vi "Finish.vi"   [LabVIEW 2019]
doc: "This VI is called just before exiting. It is expected to close I/O refnum, save collected data, etc."
uses:
  <vilib>/Rock Robotics/WPI/Utilities/WPI_GetSetVariantRefNum.vi
types:
  T1 = typedef "WPI_JoystickDevRef.ctl" = cluster{"Device":T2}
  T2 = typedef "WPI_JoystickDeviceEnum.ctl" = enum16{"USB 0", "USB 1", "USB 2", "USB 3", "USB 4", "USB 5"}
  T3 = typedef "WPI_CameraDevRef.ctl" = cluster{"Camera Address":string, "CameraStatus":errorcluster}
  T4 = typedef "WPI_SolenoidDevRef.ctl" = cluster{"DevStatus":errorcluster, "Pneumatics Control Module":u8, "Forward Solenoid Channel":T5, "Reverse Solenoid Channel":T5}
  T5 = typedef "WPI_SolenoidChannel.ctl" = enum8{"Solenoid 0", "Solenoid 1", "Solenoid 2", "Solenoid 3", "Solenoid 4", "Solenoid 5", "Solenoid 6", "Solenoid 7", "Invalid"}
  T6 = typedef "WPI_CompressorDevRef.ctl" = cluster{"DevStatus":errorcluster, "Pneumatics Control Module":u8}
  T7 = typedef "WPI_RobotDriveDevRef.ctl" = cluster{"DevStatus":errorcluster, "Motors[]":T8[], "Square Inputs":bool, "Max Output":dbl}
  T8 = typedef "WPI_MotorControlDeviceRef.ctl" = cluster{"DeviceStatus":errorcluster, "Type":T9, "PWM":cluster{"PWM Channel":T10, "DeadBand":T11}, "CAN":cluster{"Device Number":u8, "SetOutput VI Ref":variant, "GetOutput VI Ref":variant, "Enable VI Ref":variant, "Disable VI Ref":variant, "Data":variant}, "Invert":bool, "DIO PWM":cluster{"PWM \"Enable\" Channel":T10, "DIOChannel":T12, "PWM Rate":dbl}}
  T9 = typedef "WPI_MotorControlType.ctl" = enum16{"PWM", "CAN", "DIO PWM"}
  T10 = typedef "FPGA_DIOPWMChannel.ctl" = enum8{"PWM 0", "PWM 1", "PWM 2", "PWM 3", "PWM 4", "PWM 5", "PWM 6", "PWM 7", "PWM 8", "PWM 9", "PWM MXP 0", "PWM MXP 1", "PWM MXP 2", "PWM MXP 3", "PWM MXP 4", "PWM MXP 5", "PWM MXP 6", "PWM MXP 7", "PWM MXP 8", "PWM MXP 9", "Invalid"}
  T11 = typedef "WPI_PWMDeadband.ctl" = cluster{"Name":string, "maxPositivePwm":i32, "minPositivePwm":i32, "centerPwm":i32, "maxNegativePwm":i32, "minNegativePwm":i32, "angularRange":u16}
  T12 = typedef "FPGA_DIOChannel.ctl" = enum8{"DIO 0", "DIO 1", "DIO 2", "DIO 3", "DIO 4", "DIO 5", "DIO 6", "DIO 7", "DIO 8", "DIO 9", "DIO MXP 0", "DIO MXP 1", "DIO MXP 2", "DIO MXP 3", "DIO MXP 4", "DIO MXP 5", "DIO MXP 6", "DIO MXP 7", "DIO MXP 8", "DIO MXP 9", "DIO MXP 10", "DIO MXP 11", "DIO MXP 12", "DIO MXP 13", "DIO MXP 14", "DIO MXP 15", "SPI Port CS1", "SPI Port CS2", "SPI Port CS3", "SPI Port MISO", "SPI Port MOSI", "Invalid"}
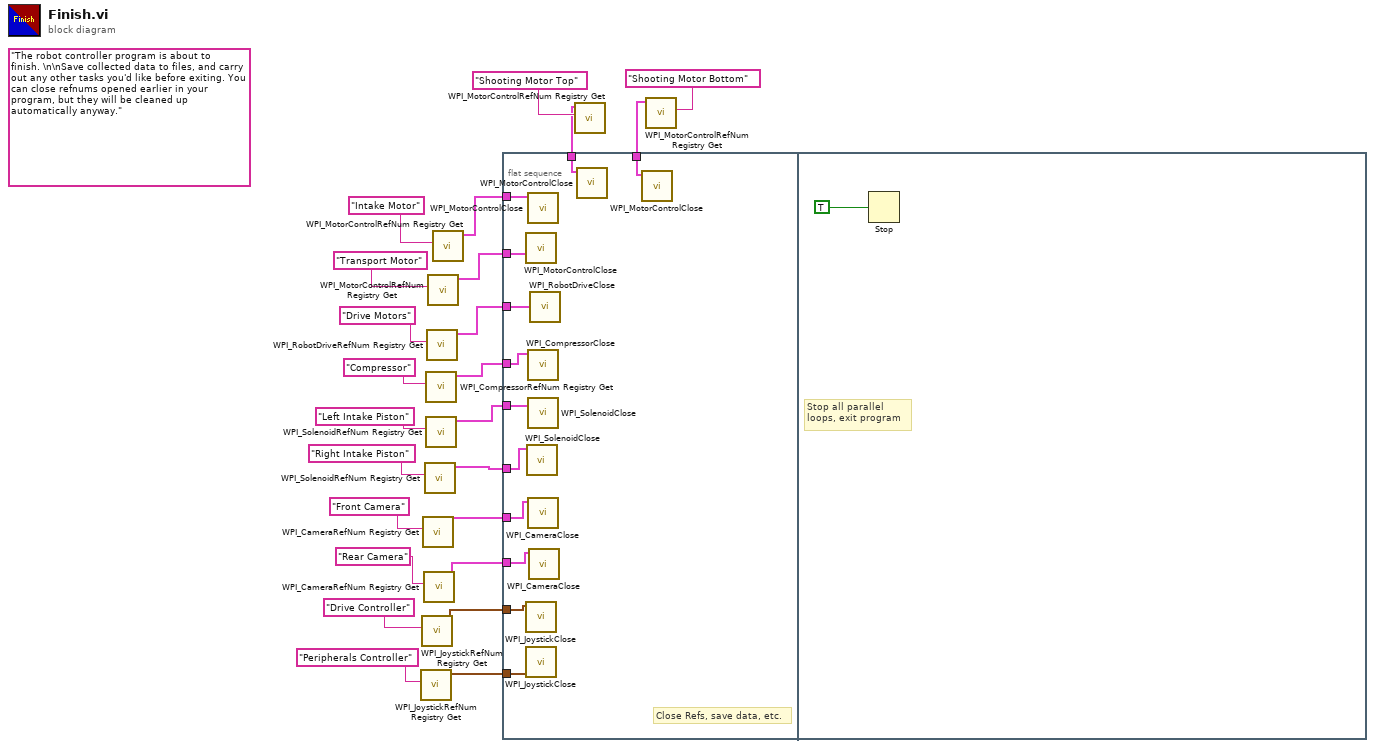
[diagram p0: block diagram]
diagram:
  (unwired) "The robot controller program is about to finish. \n\nSave collected data to files, and carry out any other tasks you'd like before exiting. You can close refnums opened earlier in your program, but they will be cleaned up automatically anyway."
  n1 = call <vilib>:"WPI_JoystickRefNum Registry Get.vi"("refnum name"="Peripherals Controller") -> ("JoystickDevRef"=w5:T1)  [unwired: 9 in, 1 out]
  n2 = call <vilib>:"WPI_JoystickRefNum Registry Get.vi"("refnum name"="Drive Controller") -> ("JoystickDevRef"=w6:T1)  [unwired: 9 in, 1 out]
  n3 = call <vilib>:"WPI_CameraRefNum Registry Get.vi"("refnum name"="Front Camera") -> ("CameraDevRef"=w9:T3)  [unwired: 9 in, 1 out]
  n4 = call <vilib>:"WPI_CameraRefNum Registry Get.vi"("refnum name"="Rear Camera") -> ("CameraDevRef"=w10:T3)  [unwired: 9 in, 1 out]
  n5 = call <vilib>:"WPI_SolenoidRefNum Registry Get.vi"("refnum name"="Right Intake Piston") -> ("SolenoidDevRef"=w15:T4)  [unwired: 9 in, 1 out]
  n6 = call <vilib>:"WPI_CompressorRefNum Registry Get.vi"("refnum name"="Compressor") -> ("CompressorDevRef"=w18:T6)  [unwired: 9 in, 1 out]
  n7 = call <vilib>:"WPI_SolenoidRefNum Registry Get.vi"("refnum name"="Left Intake Piston") -> ("SolenoidDevRef"=w16:T4)  [unwired: 9 in, 1 out]
  n8 = call <vilib>:"WPI_RobotDriveRefNum Registry Get.vi"("refnum name"="Drive Motors") -> ("RobotDriveDevRef"=w23:T7)  [unwired: 1 in, 9 out]
  n9 = call <vilib>:"WPI_MotorControlRefNum Registry Get.vi"("refnum name"="Transport Motor") -> ("MotorControlDevRef"=w19:T8)  [unwired: 9 in, 1 out]
  n10 = call <vilib>:"WPI_MotorControlRefNum Registry Get.vi"("refnum name"="Intake Motor") -> ("MotorControlDevRef"=w22:T8)  [unwired: 9 in, 1 out]
  n11 = flat-sequence {
    tunnel: w23 -> [w36]
    tunnel: w22 -> [w35]
    tunnel: w19 -> [w34]
    tunnel: w18 -> [w31]
    tunnel: w16 -> [w33]
    tunnel: w15 -> [w32]
    tunnel: w10 -> [w30]
    tunnel: w9 -> [w29]
    tunnel: w6 -> [w28]
    tunnel: w5 -> [w27]
    tunnel: w2 -> [w26]
    tunnel: w1 -> [w25]
    frame #0 {
      # "Close Refs, save data, etc."
      n12 = call <vilib>:"WPI_MotorControlClose.vi"("MotorControlDevRef"=w34) -> ()  [unwired: 10 in, 1 out]
      n13 = call <vilib>:"WPI_JoystickClose.vi"("JoystickDevRef"=w28) -> ()  [unwired: 11 in]
      n14 = call <vilib>:"WPI_JoystickClose.vi"("JoystickDevRef"=w27) -> ()  [unwired: 11 in]
      n15 = call <vilib>:"WPI_SolenoidClose.vi"("SolenoidDevRef"=w32) -> ()  [unwired: 10 in, 1 out]
      n16 = call <vilib>:"WPI_MotorControlClose.vi"("MotorControlDevRef"=w35) -> ()  [unwired: 10 in, 1 out]
      n17 = call <vilib>:"WPI_CompressorClose.vi"("CompressorDevRef"=w31) -> ()  [unwired: 10 in, 1 out]
      n18 = call <vilib>:"WPI_SolenoidClose.vi"("SolenoidDevRef"=w33) -> ()  [unwired: 10 in, 1 out]
      n19 = call <vilib>:"WPI_CameraClose.vi"("CameraDevRef"=w29) -> ()  [unwired: 10 in, 1 out]
      n20 = call <vilib>:"WPI_CameraClose.vi"("CameraDevRef"=w30) -> ()  [unwired: 10 in, 1 out]
      n21 = call <vilib>:"WPI_RobotDriveClose.vi"("RobotDriveDevRef"=w36) -> ()  [unwired: 1 in, 10 out]
      n22 = call <vilib>:"WPI_MotorControlClose.vi"("MotorControlDevRef"=w26) -> ()  [unwired: 10 in, 1 out]
      n23 = call <vilib>:"WPI_MotorControlClose.vi"("MotorControlDevRef"=w25) -> ()  [unwired: 10 in, 1 out]
    }
    frame #1 {
      # "Stop all parallel\nloops, exit program"
      n24 = Stop(stop? (T)=TRUE ("Quit")) -> ()
    }
  }
  n25 = call <vilib>:"WPI_MotorControlRefNum Registry Get.vi"("refnum name"="Shooting Motor Top") -> ("MotorControlDevRef"=w2:T8)  [unwired: 9 in, 1 out]
  n26 = call <vilib>:"WPI_MotorControlRefNum Registry Get.vi"("refnum name"="Shooting Motor Bottom") -> ("MotorControlDevRef"=w1:T8)  [unwired: 9 in, 1 out]
